vi "LCR_PlotHelper.vi"(5 "Y-Axis":T3, 7 "X-Axis":T3, 9 "Data_IN":T1, 11 "Graph REF":refnum<vi>) -> (0 "Graph Out":cluster{"Variant X":dbl, "Variant Y":dbl}[](array[cluster]), 1 "Data_Out":T1)   [LabVIEW 2021]
uses:
  Plotting-Axis.ctl
  Data_Cluster.ctl
  Measurement_Cluster.ctl
  82b2c7e2-1130-4631-9edb-692d0da541f7.vi
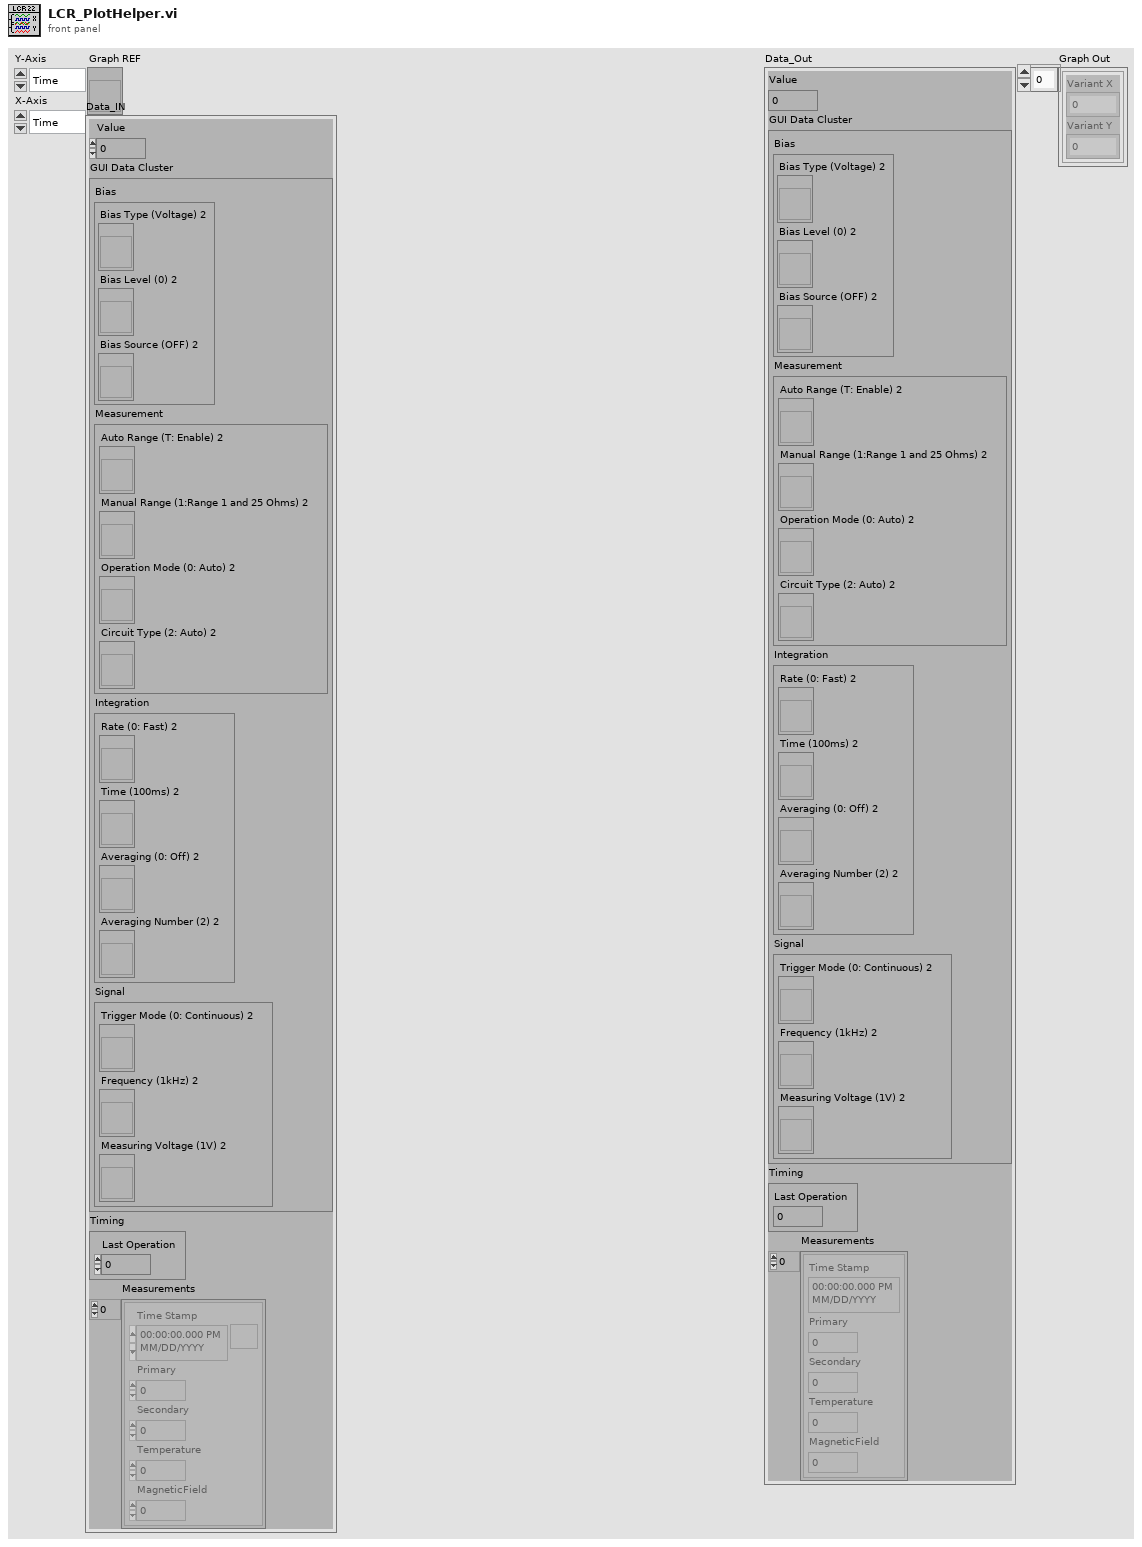
[diagram p1: front panel]
types:
  T1 = typedef "Data_Cluster.ctl" = cluster{"Value":dbl, "GUI Data Cluster":cluster{"Bias":cluster{"Bias Type (Voltage) 2":refnum<vi>, "Bias Level (0) 2":refnum<vi>, "Bias Source (OFF) 2":refnum<vi>}, "Measurement":cluster{"Auto Range (T: Enable) 2":refnum<vi>, "Manual Range (1:Range 1 and 25 Ohms) 2":refnum<vi>, "Operation Mode (0: Auto) 2":refnum<vi>, "Circuit Type (2: Auto) 2":refnum<vi>}, "Integration":cluster{"Rate (0: Fast) 2":refnum<vi>, "Time (100ms) 2":refnum<vi>, "Averaging (0: Off) 2":refnum<vi>, "Averaging Number (2) 2":refnum<vi>}, "Signal":cluster{"Trigger Mode (0: Continuous) 2":refnum<vi>, "Frequency (1kHz) 2":refnum<vi>, "Measuring Voltage (1V) 2":refnum<vi>}}, "Timing":cluster{"Last Operation":dbl}, "Measurements":T2[]}
  T2 = typedef "Measurement_Cluster.ctl" = cluster{"Time Stamp":timestamp, "Primary":dbl, "Secondary":dbl, "Temperature":dbl, "MagneticField":dbl}
  T3 = typedef "Plotting-Axis.ctl" = enum16{"Time", "Temperature", "MagneticField", "Primary", "Secondary"}
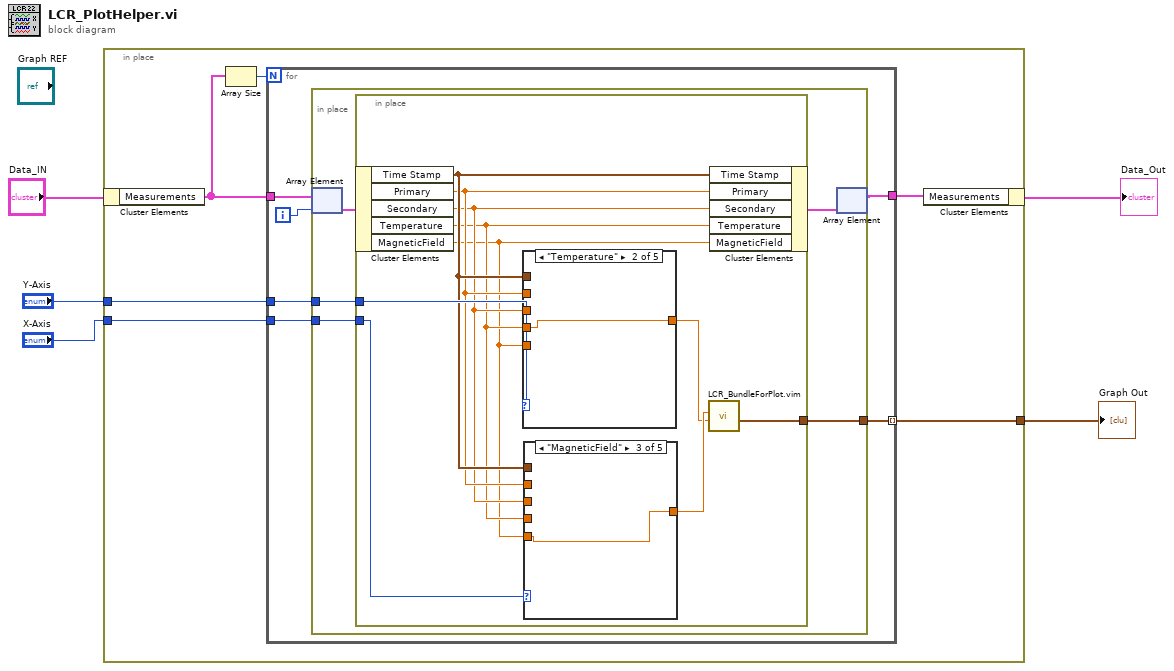
[diagram p0: block diagram]
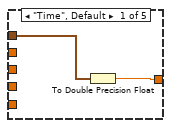
[diagram p2: hidden frame]
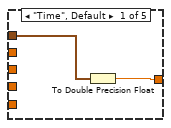
[diagram p6: hidden frame]
diagram:
  n1 = in-place {
    in-place-border: "Y-Axis" -> [w9]
    in-place-border: "X-Axis" -> [w8]
    in-place-border: [w6] -> w1
    n2 = in-place-cluster #1("Data_IN") -> ("Measurements"=w11:T2[])
    n3 = Array Size(array=w11) -> (size(s)=w10:i32)
    n4 = for {
      N: w10 -> [_]
      tunnel: w11 -> [w17]
      tunnel: w9 -> [w15]
      tunnel: w8 -> [w14]
      tunnel: [w13] -> w7
      tunnel: [w12] -> w6 mode=indexing
      i -> [w16]
      n5 = in-place {
        in-place-border: w15 -> [w21]
        in-place-border: w14 -> [w20]
        in-place-border: [w18] -> w12
        n6 = in-place-array #2(w17, w16) -> (w22:T2)
        n7 = in-place {
          in-place-border: w21 -> [w32]
          in-place-border: w20 -> [w31]
          in-place-border: [w23] -> w18
          n8 = in-place-cluster #3(w22) -> ("Time Stamp"=w28:timestamp, "Primary"=w27:dbl, "Secondary"=w26:dbl, "Temperature"=w25:dbl, "MagneticField"=w24:dbl)
          n9 = case shown="\"Temperature\"" w32 {
            tunnel: w28 -> [w40 _ _ _ _]
            tunnel: w27 -> [_ _ _ w43 _]
            tunnel: w26 -> [_ _ _ _ w44]
            tunnel: w25 -> [_ w41 _ _ _]
            tunnel: w24 -> [_ _ w42 _ _]
            tunnel: [w39 w41 w42 w43 w44] -> w29
            frame "Time", Default {
              n10 = To Double Precision Float(number=w40) -> (double precision float=w39:dbl)
            }
            frame "Temperature" {
            }
            frame "MagneticField" {
            }
            frame "Primary" {
            }
            frame "Secondary" {
            }
          }
          n11 = case shown="\"MagneticField\"" w31 {
            tunnel: w28 -> [w34 _ _ _ _]
            tunnel: w27 -> [_ _ _ w37 _]
            tunnel: w26 -> [_ _ _ _ w38]
            tunnel: w25 -> [_ w35 _ _ _]
            tunnel: w24 -> [_ _ w36 _ _]
            tunnel: [w33 w35 w36 w37 w38] -> w30
            frame "Time", Default {
              n12 = To Double Precision Float(number=w34) -> (double precision float=w33:dbl)
            }
            frame "Temperature" {
            }
            frame "MagneticField" {
            }
            frame "Primary" {
            }
            frame "Secondary" {
            }
          }
          n13 = call "LCR_BundleForPlot.vim"("Variant Y"=w29, "Variant X"=w30) -> ("Bundled Variant"=w23:cluster{"Variant X":dbl, "Variant Y":dbl})  [unwired: 9 in]
          n14 = in-place-cluster #3("Time Stamp"=w28, "Primary"=w27, "Secondary"=w26, "Temperature"=w25, "MagneticField"=w24) -> (w19:T2)
        }
        n15 = in-place-array #2(w19) -> (w13:T2[])  [unwired: 1 out]
      }
    }
    n16 = in-place-cluster #1("Measurements"=w7) -> (→"Data_Out":T1)
  }
  "Graph Out" <- w1
